vi "Configure Bit Transition Waveform.vi"(6 "Enable Interpolation (F: Disable)":bool, 7 "Values List (0)":dbl[](array[numeric]), 8 "error in (no error)":errorcluster, 9 "Bit Transition Waveform Name (CAP_2)":string, 10 "Operation (0: Download Bit Shape Waveform)":i32(ring) items=["Download Bit Shape Waveform", "Enable Interpolation", "Load Bit Shape Waveform", "Store Bit Shape Waveform", "Delete Bit Shape Waveform"], 11 "VISA resource name":refnum<visa-resource-name>) -> (0 "error out":errorcluster, 3 "VISA resource name out":refnum<visa-resource-name>)   [LabVIEW 2009, in "Agilent 81150.lvlib"]
doc: "Configures the bit shape transition waveform."
uses:
  Agilent 81150.lvlib
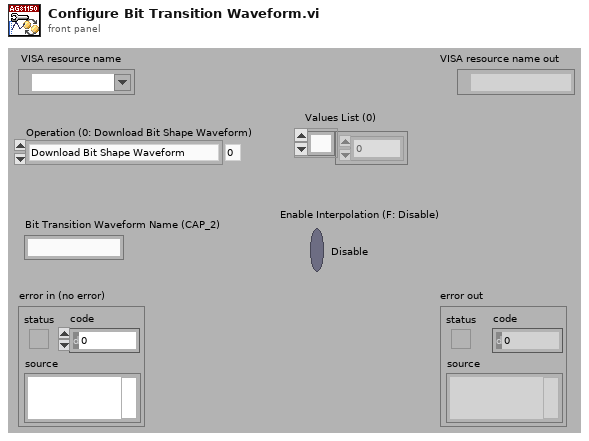
[diagram p1: front panel]
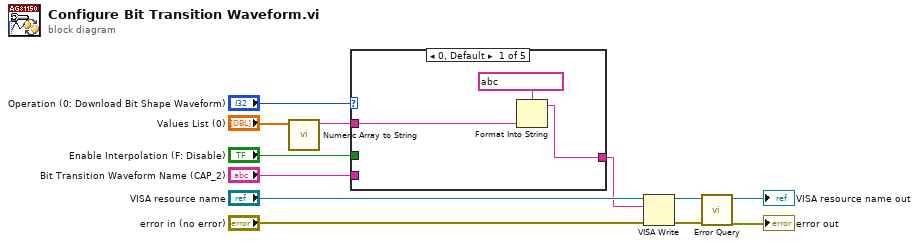
[diagram p0: block diagram]
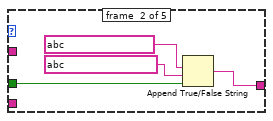
[diagram p2: hidden frame]
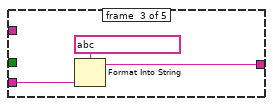
[diagram p3: hidden frame]
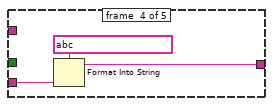
[diagram p4: hidden frame]
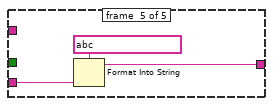
[diagram p5: hidden frame]
diagram:
  n1 = call "Numeric Array to String.vi"("List Data"="Values List (0)") -> ("Result String"=w1:string)  [unwired: 10 in]
  n2 = case shown="0, Default" "Operation (0: Download Bit Shape Waveform)" {
    tunnel: [w14 w16 w20 w23 w26] -> w5
    tunnel: "Enable Interpolation (F: Disable)" -> [_ w17 _ _ _]
    tunnel: "Bit Transition Waveform Name (CAP_2)" -> [_ _ w21 w24 w27]
    tunnel: w1 -> [w13 _ _ _ _]
    frame #0 {
      n3 = Format Into String(format string=string ?, w13) -> (resulting string=w14:string)  [unwired: 2 in, 1 out]
    }
    frame #1 {
      n4 = Append True/False String(1:w17, 2:string ?, 3:string ?) -> (0:w16:string)  [unwired: 1 in]
    }
    frame #2 {
      n5 = Format Into String(format string=string ?, w21) -> (resulting string=w20:string)  [unwired: 2 in, 1 out]
    }
    frame #3 {
      n6 = Format Into String(format string=string ?, w24) -> (resulting string=w23:string)  [unwired: 2 in, 1 out]
    }
    frame #4 {
      n7 = Format Into String(format string=string ?, w27) -> (resulting string=w26:string)  [unwired: 2 in, 1 out]
    }
  }
  n8 = VISA Write(VISA resource name="VISA resource name", write buffer=w5, error in (no error)="error in (no error)") -> (VISA resource name out=w10:refnum<visa-resource-name>, error out=w9:errorcluster)  [unwired: 1 out]
  n9 = call "Error Query.vi"("error in (no error)"=w9, "VISA resource name"=w10) -> ("error out"=→"error out":errorcluster, "VISA resource name out"=→"VISA resource name out":refnum<visa-resource-name>)  [unwired: 6 in, 2 out]
